vi "myRIO_Brig_RT__Case_Exp_State_initTrial__v2.vi"(7 "input_spout":enum16{"Left", "Right"}(ring), 8 "input_dataBlock":u16[][](array[numeric]), 10 "input_dataExp":u16[](array[numeric]), 11 "input_dataCurrent":u16[](array[numeric])) -> (1 "output_state":T1=enum."ENL1_pre", 2 "output_dataExp":u16[](array[numeric]), 3 "output_dataCurrent":u16[](array[numeric]), 4 "output_iTrial":u16, 6 "output_SolenoidReward":bool)   [LabVIEW 2014]
uses:
  myRIO_BRig_RT__Case_Exp_stateList.ctl
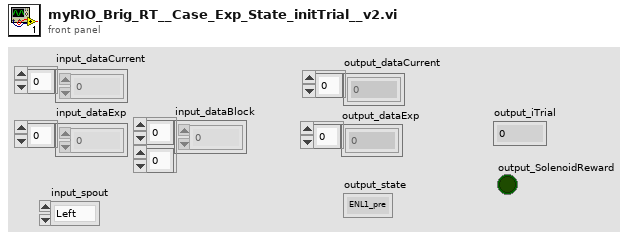
[diagram p1: front panel]
types:
  T1 = typedef "myRIO_BRig_RT__Case_Exp_stateList.ctl" = enum16{"Start1", "Start2", "Start3", "saveSettings1", "saveSettings2", "saveSettings3", "saveSettings4", "saveSettings_LC_ENL_l1", "saveSettings_LC_ENL_l2", "saveSettings_LC_Cue_l1", "saveSettings_LC_Cue_l2", "saveSettings6_LC_l1_Other", "SaveSettings6_LC_l2_Other", "setSettings_Audio", "setSettings_Laser", "initBlock_pre", "initBlock", "initBlock2", "initBlock_post", "initTrial_pre", "initTrial", "initTrial2", "initTrial3", "initTrial4", "initTrial_LC_ENL1", "initTrial_LC_Cue1", "initTrial_LC_Cue1_2", "initTrial_LC_Sel", "initTrial_post", "ENL1_pre", "ENL1", "ENL1_post", "ENL1Penalty_pre", "ENL1Penalty", "ENL2_pre", "ENL2", "ENL2Penalty_pre", "ENL2Penalty", "Cue1_pre", "Cue1", "Cue1_post", "Cue1Penalty_pre", "Cue1Penalty", "Cue2_pre", "Cue2", "Cue2Penalty_pre", "Cue2Penalty", "Selection_pre", "Selection", "Select_post", "SelectReward_pre", "SelectReward", "SelectRewardPost_pre", "SelectRewardPost", "SelectWrong_pre", "SelectWrong", "SelectWrong_post", "SelectTimeout_pre", "SelectTimeout", "SelectTimeout_post", "endTrial_pre", "endTrial1", "endTrial2", "endTrial3", "endTrial_post", "endBlock_pre", "endBlock", "endBlock_post", "endExp", "commConnect", "commUpload_pre", "commUpload_dataBlock", "commUpload_dataCurrent", "commUpload_dataExp", "commUpload_dataLC", "commUpload_dataTrial", "commUpload_post", "saveData_pre", "saveData_dataBlock", "saveData_dataCurrent", "saveData_dataExp", "saveData_dataLC", "saveData_dataTrial", "saveData_post", "empty_endBlock1", "empty_endBlock2", "empty_endTrial1", "empty_endTrial2", "empty_endTrial3", "empty_endTrial4", "empty_endTrial5", "dummyState", "dummyState_endBlock"}
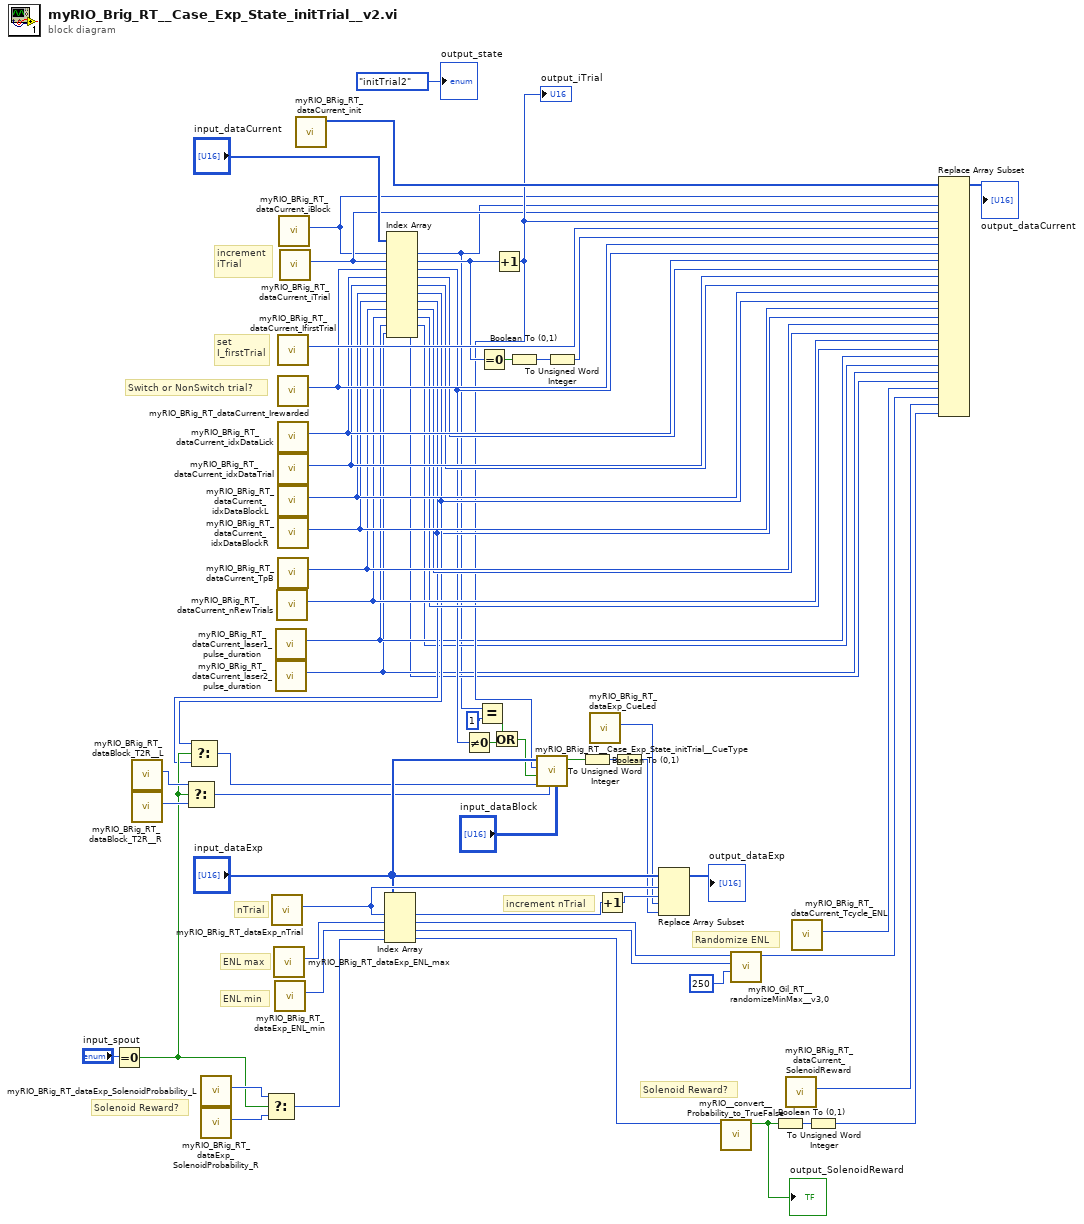
[diagram p0: block diagram]
diagram:
  # "Switch or NonSwitch trial?"
  # "Solenoid Reward?"
  # "Solenoid Reward?"
  # "ENL min"
  # "ENL max"
  # "nTrial"
  # "increment nTrial"
  # "set\nI_firstTrial"
  # "increment\niTrial"
  # "Randomize ENL"
  n1 = Equal To 0?(x="input_spout") -> (x = 0?=w26:bool)
  n2 = call "myRIO_BRig_RT_dataBlock_T2R__L.vi"() -> ("output_T2R__L"=w28:i32)  [unwired: 11 in]
  n3 = call "myRIO_BRig_RT_dataBlock_T2R__R.vi"() -> ("output_T2R__R"=w29:i32)  [unwired: 11 in]
  n4 = Select(t=w28, s=w26, f=w29) -> (s? t:f=w27:i32)
  n5 = call "myRIO_BRig_RT_dataExp_SolenoidProbability_L.vi"() -> ("output_SolenoidProbability_L"=w53:i32)  [unwired: 11 in]
  n6 = call "myRIO_BRig_RT_dataExp_SolenoidProbability_R.vi"() -> ("output_SolenoidProbability_R"=w52:i32)  [unwired: 11 in]
  n7 = Select(t=w53, s=w26, f=w52) -> (s? t:f=w44:i32)
  n8 = call "myRIO_BRig_RT_dataExp_nTrial.vi"() -> ("output_nTrial"=w59:i32)  [unwired: 11 in]
  n9 = call "myRIO_BRig_RT_dataExp_ENL_max.vi"() -> ("output_ENL_max"=w58:i32)  [unwired: 11 in]
  n10 = call "myRIO_BRig_RT_dataExp_ENL_min.vi"() -> ("output_ENL_min"=w57:i32)  [unwired: 11 in]
  n11 = call "myRIO_BRig_RT_dataCurrent_laser1_pulse_duration.vi"() -> ("output_laser1_pulse_duration"=w12:i32)  [unwired: 11 in]
  n12 = call "myRIO_BRig_RT_dataCurrent_laser2_pulse_duration.vi"() -> ("output_laser2_pulse_duration"=w11:i32)  [unwired: 11 in]
  n13 = call "myRIO_BRig_RT_dataCurrent_nRewTrials.vi"() -> ("output_nRewTrials"=w32:i32)  [unwired: 11 in]
  n14 = call "myRIO_BRig_RT_dataCurrent_IfirstTrial.vi"() -> ("output_I_firstTrial"=w63:i32)  [unwired: 11 in]
  n15 = call "myRIO_BRig_RT_dataCurrent_Irewarded.vi"() -> ("output_I_rewarded"=w43:i32)  [unwired: 11 in]
  n16 = call "myRIO_BRig_RT_dataCurrent_idxDataLick.vi"() -> ("output_idxDataLick"=w40:i32)  [unwired: 11 in]
  n17 = call "myRIO_BRig_RT_dataCurrent_idxDataTrial.vi"() -> ("output_idxDataTrial"=w38:i32)  [unwired: 11 in]
  n18 = call "myRIO_BRig_RT_dataCurrent_idxDataBlockL.vi"() -> ("output_idxDataBlock__L"=w36:i32)  [unwired: 11 in]
  n19 = call "myRIO_BRig_RT_dataCurrent_idxDataBlockR.vi"() -> ("output_idxDataBlock__R"=w35:i32)  [unwired: 11 in]
  n20 = call "myRIO_BRig_RT_dataCurrent_TpB.vi"() -> ("output_TpB"=w34:i32)  [unwired: 11 in]
  n21 = call "myRIO_BRig_RT_dataCurrent_iBlock.vi"() -> ("output_iBlock"=w6:i32)  [unwired: 11 in]
  n22 = call "myRIO_BRig_RT_dataCurrent_iTrial.vi"() -> ("output_iTrial"=w7:i32)  [unwired: 11 in]
  n23 = call "myRIO_BRig_RT_dataCurrent_init.vi"() -> ("output_dataCurrent"=w45:u16[])  [unwired: 11 in]
  n24 = Index Array(array="input_dataExp", index #1=w59, index #2=w58, index #3=w57, index #4=w44) -> (element #1=w56:u16, element #2=w55:u16, element #3=w54:u16, element #4=w42:u16)
  n25 = Index Array(array="input_dataCurrent", index #1=w6, index #2=w7, index #3=w43, index #4=w40, index #5=w38, index #6=w36, index #7=w35, index #8=w34, index #9=w32, index #10=w12, index #11=w11) -> (element #1=w2:u16, element #2=w49:u16, element #3=w22:u16, element #4=w39:u16, element #5=w37:u16, element #6=w25:u16, element #7=w24:u16, element #8=w33:u16, element #9=w31:u16, element #10=w10:u16, element #11=w9:u16)
  n26 = Select(t=w25, s=w26, f=w24) -> (s? t:f=w23:u16)
  n27 = Not Equal To 0?(x=w22) -> (x != 0?=w5:bool)
  n28 = Equal?(x=w2, y=u16 1) -> (x = y?=w3:bool)
  n29 = Equal To 0?(x=w49) -> (x = 0?=w48:bool)
  n30 = Or(x=w3, y=w5) -> (x .or. y?=w4:bool)
  n31 = Increment(x=w49) -> (x+1=w21:u16)
  "output_iTrial" <- w21
  n32 = Boolean To (0,1)(Boolean=w48) -> (0, 1=w47:i16)
  n33 = call "myRIO_BRig_RT__Case_Exp_State_initTrial__CueType.vi"("input_dataBlock"="input_dataBlock", "input_idxDataBlock_T2R"=w27, "input_idxDataBlock"=w23, "input_I_reward"=w4, "input_iTrial"=w21, "input_dataExp"="input_dataExp") -> ("output_LED"=w8:bool)  [unwired: 5 in]
  n34 = To Unsigned Word Integer(number=w47) -> (unsigned 16bit integer=w46:u16)
  n35 = Boolean To (0,1)(Boolean=w8) -> (0, 1=w18:i16)
  n36 = call "myRIO_BRig_RT_dataExp_CueLed.vi"() -> ("output_CueLed"=w19:i32)  [unwired: 11 in]
  n37 = Increment(x=w56) -> (x+1=w62:u16)
  n38 = To Unsigned Word Integer(number=w18) -> (unsigned 16bit integer=w17:u16)
  n39 = Replace Array Subset(array="input_dataExp", new element #1=w62, index #1=w59, new element #2=w17, index #2=w19) -> (→"output_dataExp":u16[])
  n40 = call "myRIO__convert__Probability_to_TrueFalse.vi"("input_probability_u16"=w42) -> ("output_TF"=w41:bool)  [unwired: 10 in]
  "output_SolenoidReward" <- w41
  n41 = call "myRIO_Gil_RT__randomizeMinMax__v3,0.vi"("Input_Increment"=u16 250, "Input_Min"=w54, "Input_Max"=w55) -> ("Output"=w15:u16)  [unwired: 8 in]
  n42 = Boolean To (0,1)(Boolean=w41) -> (0, 1=w50:i16)
  n43 = call "myRIO_BRig_RT_dataCurrent_SolenoidReward.vi"() -> ("output_SolenoidReward"=w14:i32)  [unwired: 11 in]
  n44 = call "myRIO_BRig_RT_dataCurrent_Tcycle_ENL.vi"() -> ("output_ENL"=w16:i32)  [unwired: 11 in]
  n45 = To Unsigned Word Integer(number=w50) -> (unsigned 16bit integer=w13:u16)
  n46 = Replace Array Subset(array=w45, new element #1=w2, index #1=w6, new element #2=w21, index #2=w7, new element #3=w46, index #3=w63, new element #4=w22, index #4=w43, new element #5=w39, index #5=w40, new element #6=w37, index #6=w38, new element #7=w25, index #7=w36, new element #8=w24, index #8=w35, new element #9=w33, index #9=w34, new element #10=w31, index #10=w32, new element #11=w10, index #11=w12, new element #12=w9, index #12=w11, new element #13=w15, index #13=w16, new element #14=w13, index #14=w14) -> (→"output_dataCurrent":u16[])
  "output_state" <- myRIO_BRig_RT__Case_Exp_stateList."initTrial2" ("Enum")
